vi "Next Step.vi"(8 "error in (no error)":errorcluster, 11 "Translation Stage Fine in":refnum<class "Translation Stage Fine.lvclass">) -> (0 "error out":errorcluster, 1 "Current Step":u32, 2 "Current Position":dbl, 3 "Translation Stage Fine out":refnum<class "Translation Stage Fine.lvclass">)   [LabVIEW 2017, in "Translation Stage Fine.lvclass"]
doc: "(Dynamic) Move to the next preconfigured step of this Scanner, and return the current position (actual, not intended) of this Scanner. Increment the step counter by one."
uses:
  Translation Stage Fine.lvclass
  Global/GPIB Numbers.vi
  Scanner/Scanner.lvclass
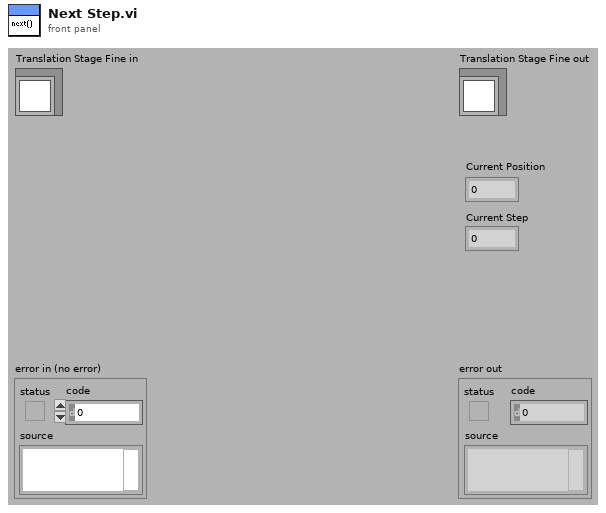
[diagram p1: front panel]
types:
  T1 = typedef "GPIB Type Def.ctl" = cluster{"Name":string, "bus":dbl, "GPIB":dbl, "GPIB as string":string, "byte":i32, "VISA Resource Name":refnum<visa-resource-name>}
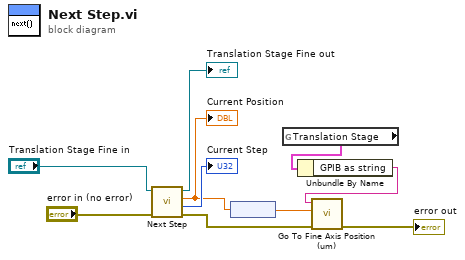
[diagram p0: block diagram]
diagram:
  n1 = call-parent "Next Step.vi"("error in (no error)"="error in (no error)", "Scanner in"="Translation Stage Fine in") -> ("error out"=w2:errorcluster, "Current Step"=→"Current Step":u32, "Current Position"=w5:dbl, "Scanner out"=→"Translation Stage Fine out":refnum<class "Translation Stage Fine.lvclass">)  [unwired: 6 in]
  "Current Position" <- w5
  n2 = node(w5) -> (w6:dbl[unit])
  n3 = global read "GPIB Numbers.vi" "Translation Stage"() -> (w4:T1)
  n4 = Unbundle By Name(w4) -> ("GPIB as string"=w3:string)
  n5 = call "Go To Fine Axis Position (um).vi"("error in"=w2, "Fine Axis Position (um)"=w6, "GPIB # (in): def. 6"=w3) -> ("error out"=→"error out":errorcluster)  [unwired: 7 in, 1 out]
